vi "Read Trace.vi"(0 "VISA resource name":refnum<visa-resource-name>, 5 "Data (0:Positive)":i32(ring) items=["Positive", "Negative"], 7 "Trace (0:Trace A)":i32(ring) items=["Trace A", "Trace B", "Trace C", "Trace D", "Trace E", "Trace F"], 9 "Start Position (0)":i32 min=0 max=10000, 11 "error in (no error)":errorcluster, 12 "Length (5001)":i32=5001 min=1 max=10001) -> (4 "VISA resource name out":refnum<visa-resource-name>, 6 "Trace Data Output":dbl[](array[numeric]), 15 "error out":errorcluster)   [LabVIEW 2020, in "Anritsu Signal Analyzer Series.lvlib"]
doc: "Reads the trace data.\n\nTargets positive detection trace data when detection mode is Positive & Negative(Normal).\nTargets negative detection trace data when detection mode is Positive & Negative(Normal)."
uses:
  Anritsu Signal Analyzer Series.lvlib
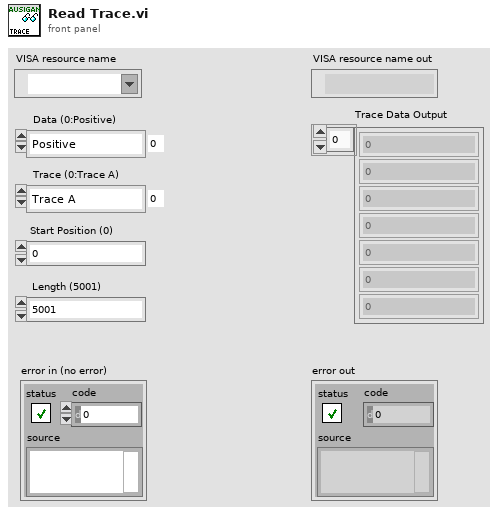
[diagram p1: front panel]
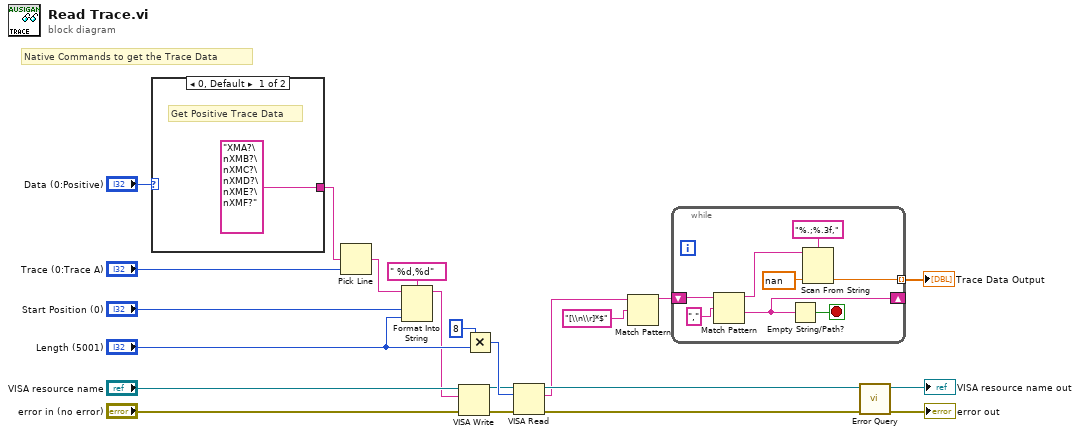
[diagram p0: block diagram]
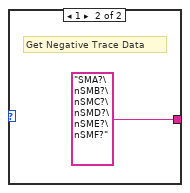
[diagram p2: hidden frame]
diagram:
  # "Native Commands to get the Trace Data"
  n1 = case shown="0, Default" "Data (0:Positive)" {
    tunnel: ["XMA?\nXMB?\nXMC?\nXMD?\nXME?\nXMF?" ("_CommandGet") "SMA?\nSMB?\nSMC?\nSMD?\nSME?\nSMF?" ("_CommandGet")] -> w9
    frame 0, Default {
      # "Get Positive Trace Data"
    }
    frame 1 {
      # "Get Negative Trace Data"
    }
  }
  n2 = Pick Line(multi-line string=w9, line index="Trace (0:Trace A)") -> (output string=w3:string)  [unwired: 1 in]
  n3 = Format Into String(format string=" %d,%d", initial string=w3, "Start Position (0)", "Length (5001)") -> (resulting string=w2:string)  [unwired: 1 in, 1 out]
  n4 = VISA Write(VISA resource name="VISA resource name", write buffer=w2, error in (no error)="error in (no error)") -> (VISA resource name out=w4:refnum<visa-resource-name>, error out=w5:errorcluster)  [unwired: 1 out]
  n5 = Multiply(x=8, y="Length (5001)") -> (x*y=w8:i32)
  n6 = VISA Read(VISA resource name=w4, byte count=w8, error in (no error)=w5) -> (VISA resource name out=w13:refnum<visa-resource-name>, read buffer=w10:string, error out=w14:errorcluster)  [unwired: 1 out]
  n7 = Match Pattern(string=w10, regular expression="[\\n\\r]*$") -> (before substring=w12:string)  [unwired: 1 in, 3 out]
  n8 = while {
    shift-right: [w25] -> _
    shift-left: w12 -> [w27]
    tunnel: [w31] -> w17 mode=indexing
    stop <- w30 stop-if-true
    n9 = Match Pattern(string=w27, regular expression=",") -> (before substring=w26:string, after substring=w25:string)  [unwired: 1 in, 2 out]
    n10 = Empty String/Path?(string/path=w25) -> (empty?=w30:bool)
    n11 = Scan From String(format string="%.;%.3f," ("Format String"), input string=w26, default 1=nan ("default value 1")) -> (output 1=w31:dbl)  [unwired: 2 in, 3 out]
  }
  "Trace Data Output" <- w17
  n12 = call "Error Query.vi"("error in (no error)"=w14, "VISA resource name"=w13) -> ("error out"=→"error out":errorcluster, "VISA resource name out"=→"VISA resource name out":refnum<visa-resource-name>)  [unwired: 6 in, 2 out]
